vi "DAQmx.Calibrate.vi"(8 "error in (no error)":errorcluster, 11 "DAQmx in":refnum<class "DAQmx.lvclass">) -> (0 "error out":errorcluster, 2 "Calibration out":T1(array[cluster]), 3 "DAQmx out":refnum<class "DAQmx.lvclass">)   [LabVIEW 2019, in "DAQmx.lvclass"]
uses:
  DAQmx.lvclass
  <vilib>/addons/WireFlow/_WF_ProgressBar.llb/WindowBehavior.ctl
  969f3a50-2d64-4ea1-bb3c-ff99df6d08b5.vi
  <vilib>/addons/WireFlow/_WF_ProgressBar.llb/ProgressBar_WireFlow.lvclass
  <resource>/objmgr/daqmx.rc
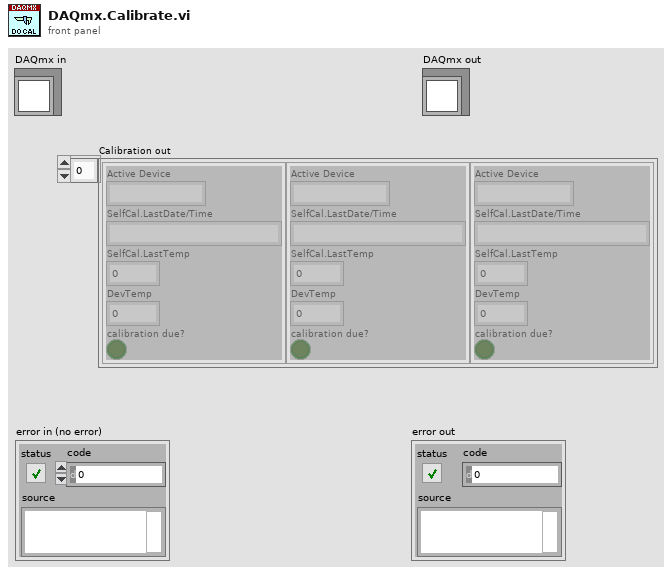
[diagram p1: front panel]
types:
  T1 = cluster{"Active Device":string, "SelfCal.LastDate/Time":string, "SelfCal.LastTemp":dbl, "DevTemp":dbl, "calibration due?":bool}[]
  T2 = typedef "ProgressBar_WireFlow.lvclass/WindowBehavior.ctl" = enum16{"No change", "Modal", "Floating"}
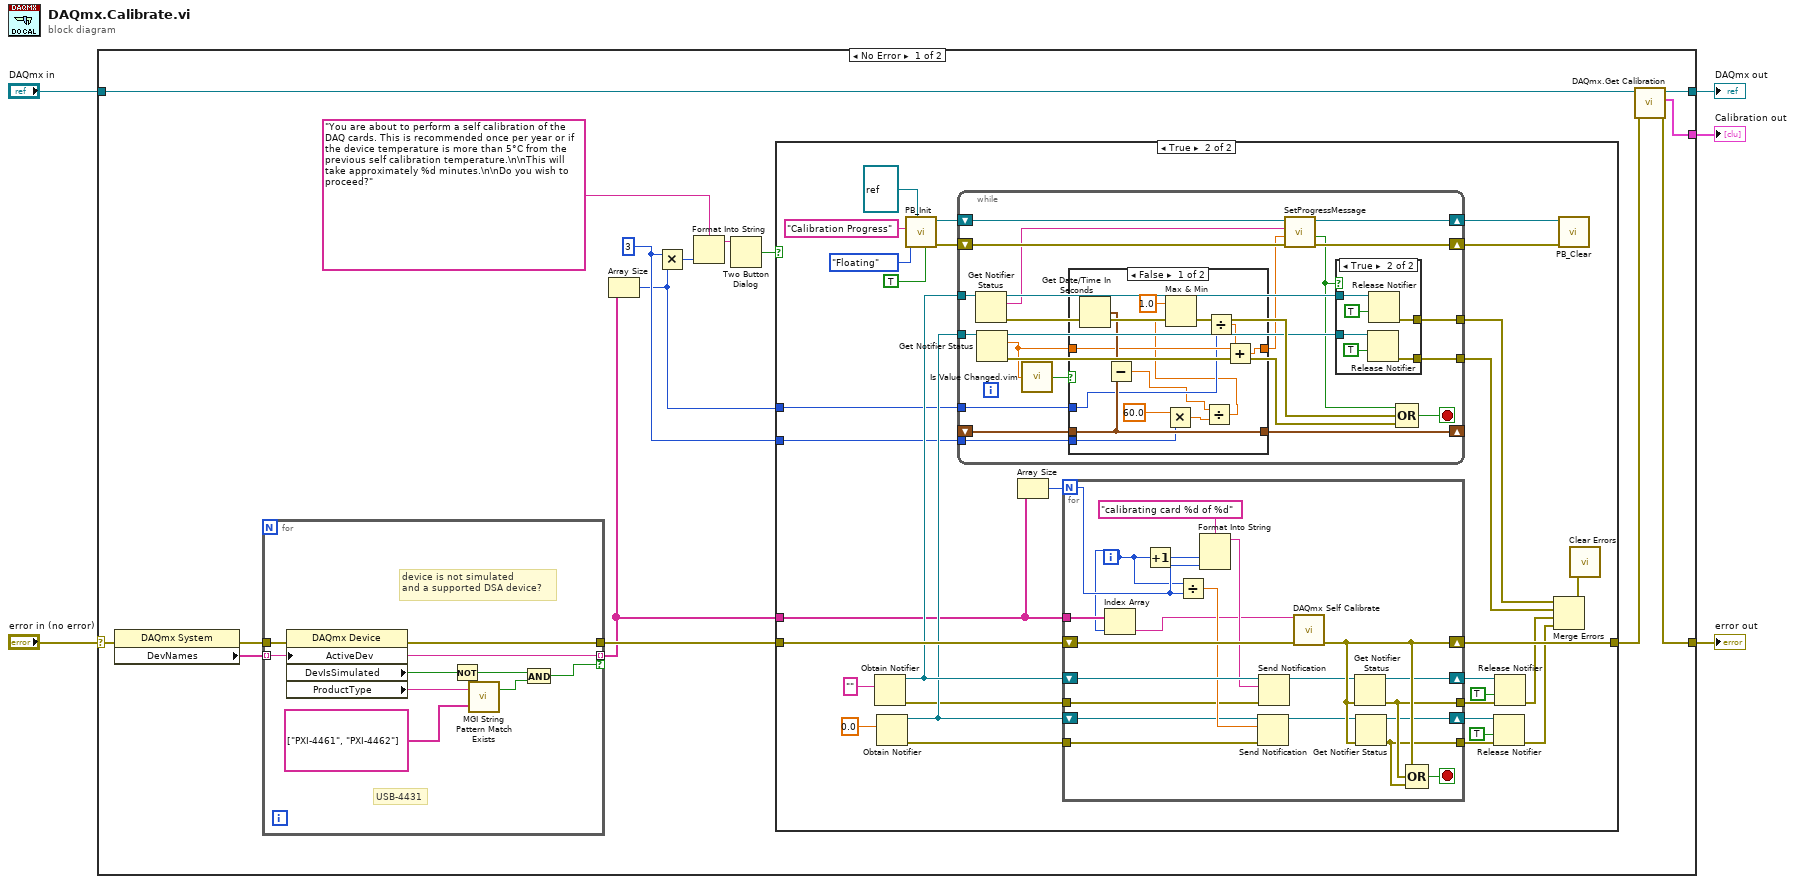
[diagram p0: block diagram]
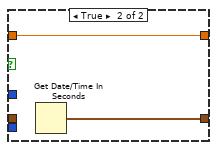
[diagram p3: hidden frame]
diagram:
  n1 = case shown="No Error" "error in (no error)" {
    selector: "error in (no error)" -> [w10 w128]
    tunnel: [w17 w127] -> w5
    tunnel: [w20 w128] -> w4
    tunnel: "DAQmx in" -> [w18 w127]
    tunnel: [w9 _] -> w2
    frame No Error {
      w7 = 3 ("x")
      n2 = property class="DAQmx System"(error in=w10) -> (error out=w15:errorcluster, "DevNames"=w16:tag[])  [unwired: 1 in, 1 out]
      n3 = for {
        tunnel: [w25] -> w13 mode=indexing if=w23
        tunnel: w16 -> [w25] mode=indexing
        tunnel: w15 -> [w24]
        tunnel: [w22] -> w14
        # "USB-4431"
        # "device is not simulated\nand a supported DSA device?"
        n4 = property class="DAQmx Device"(error in=w24, "ActiveDev"=w25) -> (error out=w22:errorcluster, "DevIsSimulated"=w30:bool, "ProductType"=w27:string)  [unwired: 1 in, 1 out]
        n5 = Not(x=w30) -> (.not. x?=w29:bool)
        n6 = call <userlib>:"MGI String Pattern Match Exists.vi"("Patterns to Try"=string[] ["PXI-4461", "PXI-4462"], "String"=w27) -> ("Match Found"=w26:bool)  [unwired: 1 out]
        n7 = And(x=w29, y=w26) -> (x .and. y?=w23:bool)
      }
      n8 = Array Size(array=w13) -> (size(s)=w6:i32)
      n9 = Multiply(x=w7, y=w6) -> (x*y=w12:i32)
      n10 = Format Into String(format string="You are about to perform a self calibration of the DAQ cards. This is recommended once per year or if the device temperature is more than 5°C from the previous self calibration temperature.\n\nThis will take approximately %d minutes.\n\nDo you wish to proceed?" ("message"), w12) -> (resulting string=w11:string)  [unwired: 2 in, 1 out]
      n11 = Two Button Dialog(message=w11) -> (T button?=w21:bool)  [unwired: 2 in]
      n12 = case shown="True" w21 {
        tunnel: w14 -> [w31 w62]
        tunnel: [w31 w61] -> w19
        tunnel: w13 -> [_ w34]
        tunnel: w7 -> [_ w40]
        tunnel: w6 -> [_ w39]
        frame False {
        }
        frame True {
          n13 = Obtain Notifier(notification data type="") -> (notifier out=w54:refnum<notifier>, error out=w47:errorcluster)  [unwired: 3 in, 1 out]
          n14 = Obtain Notifier(notification data type=0.0) -> (notifier out=w51:refnum<notifier>, error out=w48:errorcluster)  [unwired: 3 in, 1 out]
          n15 = call <vilib>:"PB_Init.vi"("Cancel button active? (False)"=TRUE, "Progress VI"=refnum<vi> refnum, "Window behavior (No change)"=WindowBehavior."Floating", "title (\"Progress\")"="Calibration Progress" ("title (\"Progress\")")) -> ("error out"=w57:errorcluster, "WF-ProgressBar out"=w58:refnum<class "ProgressBar_WireFlow.lvclass">)  [unwired: 6 in]
          n16 = while {
            shift-right: [w81] -> w59
            shift-left: w57 -> [w84]
            shift-right: [w82] -> w60
            shift-left: w58 -> [w83]
            tunnel: w54 -> [w80]
            tunnel: w51 -> [w79]
            tunnel: [w72] -> w44
            tunnel: [w71] -> w43
            shift-right: [w67] -> _
            shift-left: _ -> [w66]
            tunnel: w40 -> [w65]
            tunnel: w39 -> [w64]
            stop <- w77 stop-if-true
            n17 = Get Notifier Status(notifier=w80) -> (notifier out=w74:refnum<notifier>, current notification=w63:string, error out=w78:errorcluster)  [unwired: 1 in, 2 out]
            n18 = Get Notifier Status(notifier=w79) -> (notifier out=w75:refnum<notifier>, current notification=w68:dbl, error out=w76:errorcluster)  [unwired: 1 in, 2 out]
            n19 = call "Is Value Changed.vim"("value"=w68) -> ("changed or first call?"=w70:bool)
            n20 = case shown="False" w70 {
              tunnel: [w90 w99] -> w69
              tunnel: w68 -> [w93 w99]
              tunnel: [w96 w98] -> w67
              tunnel: w66 -> [w96 _]
              tunnel: w65 -> [w88 _]
              tunnel: w64 -> [w87 _]
              frame False {
                n21 = Get Date/Time In Seconds() -> (seconds since 1Jan1904=w97:timestamp)
                n22 = Subtract(x=w97, y=w96) -> (x-y=w85:dbl)
                n23 = Multiply(x=60.0, y=w88) -> (x*y=w94:dbl)
                n24 = Divide(x=w85, y=w94) -> (x/y=w86:dbl)
                n25 = Max & Min(x=1.0, y=w86) -> (min(x,y)=w91:dbl)  [unwired: 1 out]
                n26 = Divide(x=w91, y=w87) -> (x/y=w89:dbl)
                n27 = Add(x=w93, y=w89) -> (x+y=w90:dbl)
              }
              frame True {
                n28 = Get Date/Time In Seconds() -> (seconds since 1Jan1904=w98:timestamp)
              }
            }
            n29 = call-dynamic "SetProgressMessage.vi"("error in (no error)"=w84, "Progress value (NaN no update)"=w69, "Message"=w63, "WF-ProgressBar in"=w83) -> ("error out"=w81:errorcluster, "cancelled?"=w73:bool, "WF-ProgressBar out"=w82:refnum<class "ProgressBar_WireFlow.lvclass">)  [unwired: 5 in]
            n30 = case shown="True" w73 {
              tunnel: w75 -> [_ w104]
              tunnel: w74 -> [_ w105]
              tunnel: [_ w101] -> w71
              tunnel: [_ w100] -> w72
              frame False {
              }
              frame True {
                n31 = Release Notifier(notifier=w104, force destroy? (F)=TRUE) -> (error out=w100:errorcluster)  [unwired: 1 in, 2 out]
                n32 = Release Notifier(notifier=w105, force destroy? (F)=TRUE) -> (error out=w101:errorcluster)  [unwired: 1 in, 2 out]
              }
            }
            n33 = Compound Arithmetic op=OR(w73, w78, w76) -> (w77:bool)
          }
          n34 = Array Size(array=w34) -> (size(s)=w35:i32)
          n35 = for {
            N: w35 -> [w109]
            tunnel: w34 -> [w107]
            shift-right: [w116] -> w61
            shift-left: w62 -> [w126]
            tunnel: w48 -> [w119]
            tunnel: w47 -> [w118]
            tunnel: [w113] -> w46
            tunnel: [w112] -> w45
            shift-right: [w111] -> w50
            shift-left: w54 -> [w123]
            shift-right: [w110] -> w49
            shift-left: w51 -> [w120]
            i -> [w106]
            stop <- w117 stop-if-true
            n36 = Index Array(array=w107, index=w106) -> (element=w108:tag)
            n37 = Increment(x=w106) -> (x+1=w124:i32)
            n38 = Divide(x=w106, y=w109) -> (x/y=w121:dbl)
            n39 = Format Into String(format string="calibrating card %d of %d", w124, w109) -> (resulting string=w122:string)  [unwired: 2 in, 1 out]
            n40 = Send Notification(notification=w121, notifier=w120, error in (no error)=w119) -> (notifier out=w114:refnum<notifier>)  [unwired: 1 out]
            n41 = Send Notification(notification=w122, notifier=w123, error in (no error)=w118) -> (notifier out=w115:refnum<notifier>)  [unwired: 1 out]
            n42 = call <vilib>:"DAQmx Self Calibrate.vi"("device in"=w108, "error in"=w126) -> ("error out"=w116:errorcluster)  [unwired: 13 in]
            n43 = Get Notifier Status(notifier=w115, error in (no error)=w116) -> (notifier out=w111:refnum<notifier>, error out=w113:errorcluster)  [unwired: 3 out]
            n44 = Get Notifier Status(notifier=w114, error in (no error)=w116) -> (notifier out=w110:refnum<notifier>, error out=w112:errorcluster)  [unwired: 3 out]
            n45 = Compound Arithmetic op=OR(w116, w113, w112) -> (w117:bool)
          }
          n46 = Release Notifier(notifier=w49, force destroy? (F)=TRUE, error in (no error)=w45) -> (error out=w41:errorcluster)  [unwired: 2 out]
          n47 = Release Notifier(notifier=w50, force destroy? (F)=TRUE, error in (no error)=w46) -> (error out=w42:errorcluster)  [unwired: 2 out]
          n48 = Merge Errors(w43, w44, w42, w41) -> (w38:errorcluster)
          n49 = call-dynamic "PB_Clear.vi"("error in (no error)"=w59, "WF-ProgressBar in"=w60) -> ()  [unwired: 8 in, 2 out]
          n50 = call <vilib>:"Clear Errors.vi"("error in (no error)"=w38) -> ()  [unwired: 5 in, 2 out]
        }
      }
      n51 = call "DAQmx.Get Calibration.vi"("error in (no error)"=w19, "DAQmx in"=w18) -> ("error out"=w20:errorcluster, "Calibration out"=w9:T1, "DAQmx out"=w17:refnum<class "DAQmx.lvclass">)  [unwired: 7 in]
    }
    frame Error {
    }
  }
  "error out" <- w4
  "Calibration out" <- w2
  "DAQmx out" <- w5
